vi "Module (Top Level).vi"(8 "error in":errorcluster) -> (0 "error out":errorcluster)   [LabVIEW 2017, in "Logger.lvlib"]
uses:
  Logger.lvlib
  User Events/TypeDefs/Shutdown UE FGV Command.ctl
  Global TypeDefs/Registered Modules.ctl
  Private TypeDefs/Messages.ctl
  Error Handler/Error Handler.lvlib
panel:
  out "Log (temporary)":string
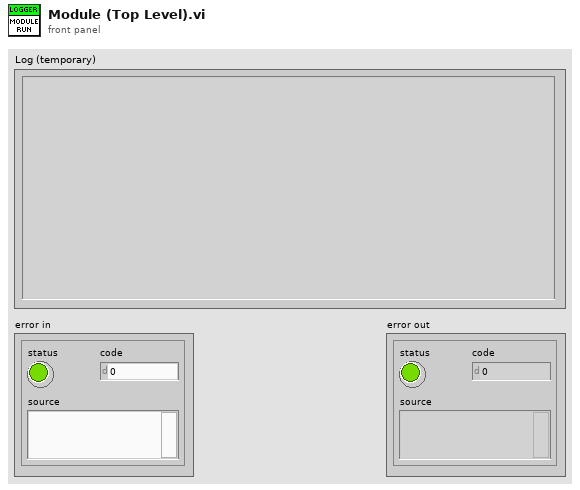
[diagram p1: front panel]
types:
  T1 = typedef "Registered Modules.ctl" = enum16{"Controller", "DAQ", "Error Handler", "Game", "myPAM", "WinHost", "Logger"}
  T2 = typedef "Shutdown UE FGV Command.ctl" = enum16{"create", "get", "destroy"}
  T3 = typedef "Logger.lvlib/Module Reference.ctl" = cluster{"calling module":T1, "module queues":T4, "module notifiers":T5}
  T4 = typedef "Logger.lvlib/Module Queues.ctl" = cluster{"message queue":refnum<queue>}
  T5 = typedef "Logger.lvlib/Module Notifiers.ctl" = cluster{"dummy notifier":refnum<notifier>}
  T6 = typedef "Error Handler.lvlib/Module Reference.ctl" = cluster{"calling module":T1, "module queues":T7, "module notifiers":T8}
  T7 = typedef "Error Handler.lvlib/Module Queues.ctl" = cluster{"message queue":refnum<queue>}
  T8 = typedef "Error Handler.lvlib/Module Notifiers.ctl" = cluster{"dummy notifier":refnum<notifier>}
  T9 = enum16{"open", "replace", "create", "open or create", "replace or create", "replace or create with confirmation"}
  T10 = typedef "Logger.lvlib/Messages.ctl" = enum16{"log event", "shutdown"}
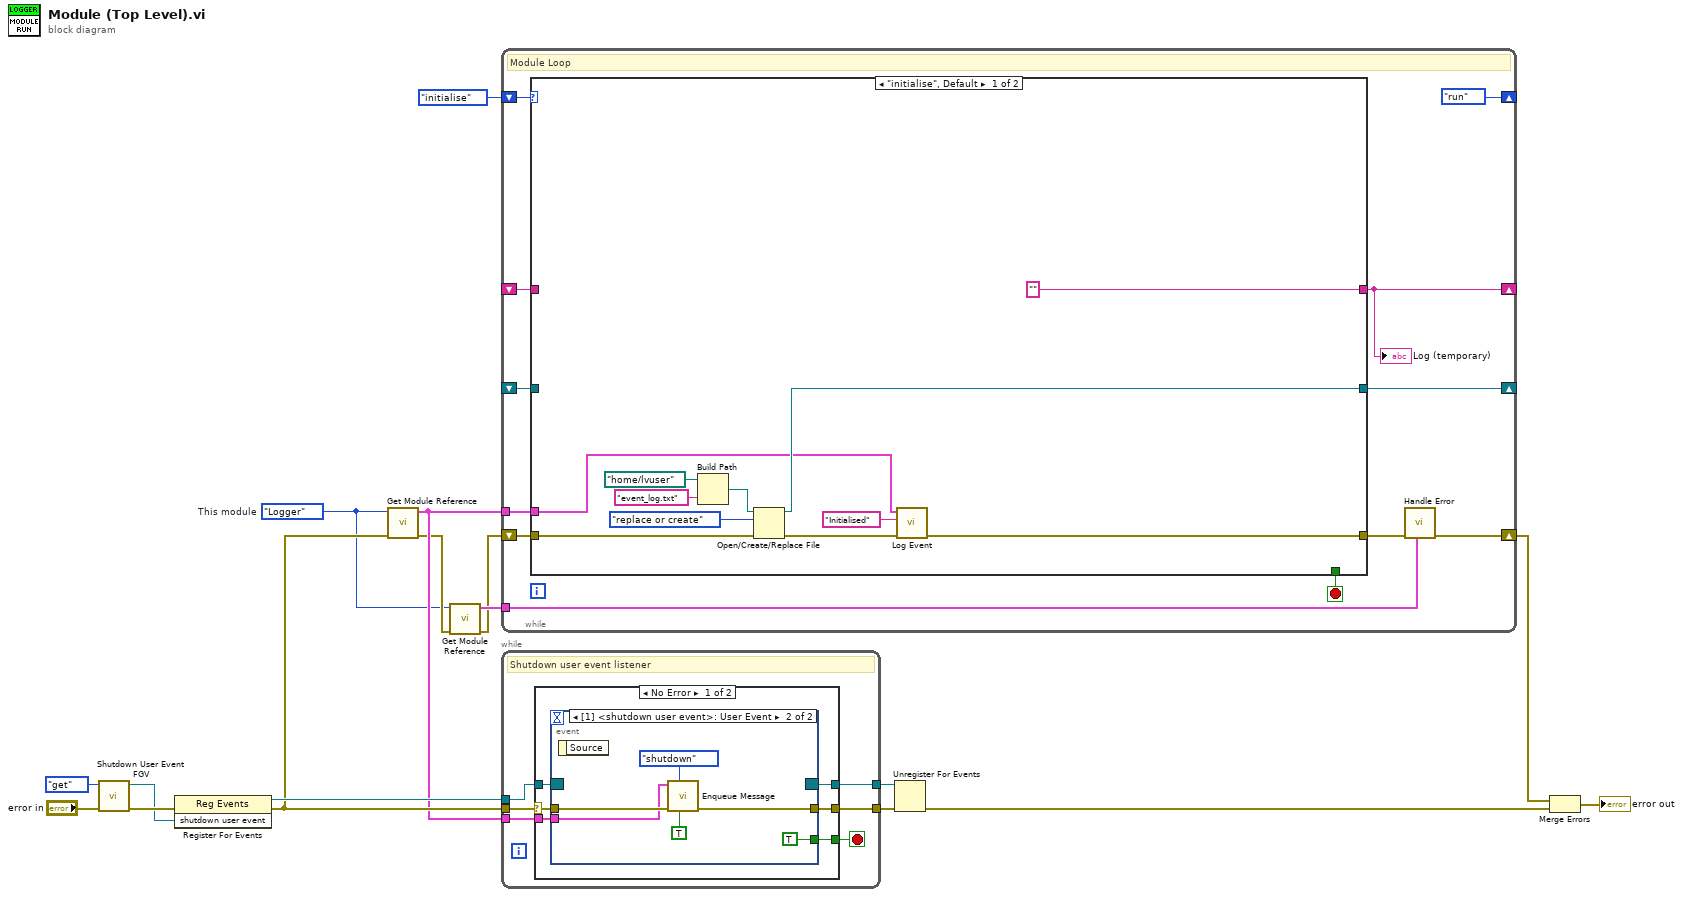
[diagram p0: block diagram]
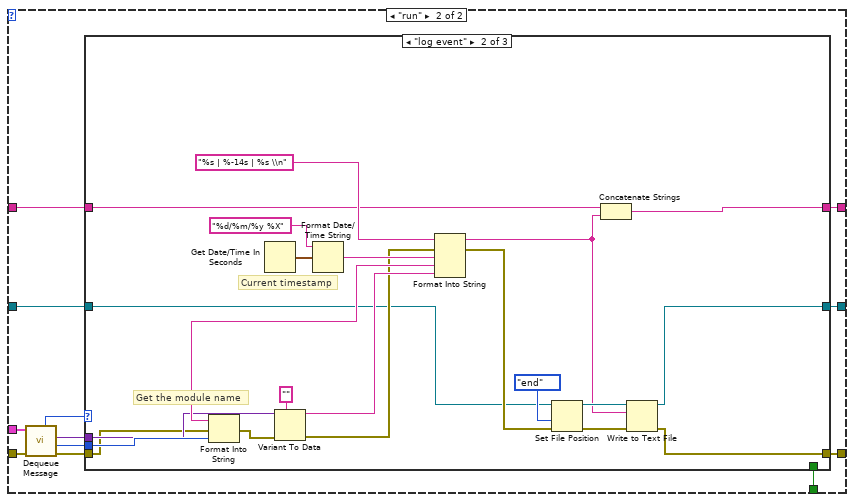
[diagram p2: hidden frame]
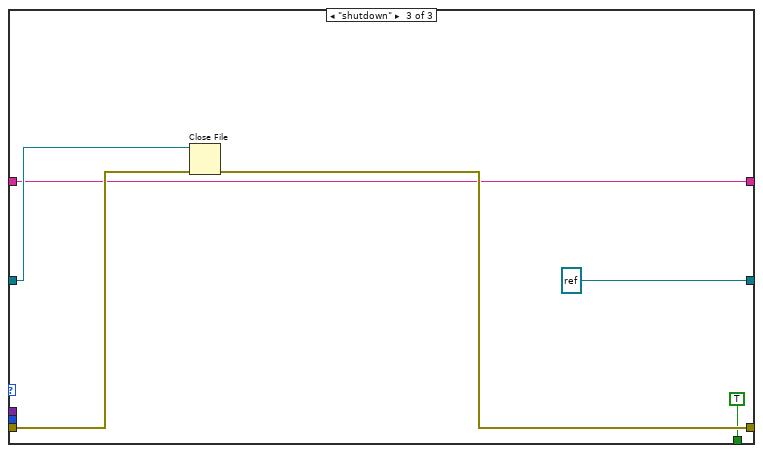
[diagram p4: hidden frame]
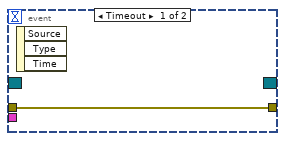
[diagram p5: hidden frame]
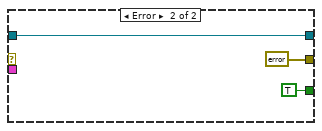
[diagram p6: hidden frame]
diagram:
  w3 = Registered_Modules."Logger"  # This module
  n1 = call "Shutdown User Event FGV.vi"("error in"="error in", "command"=Shutdown_UE_FGV_Command."get" ("Command")) -> ("error out"=w12:errorcluster, "shutdown user event"=w11:refnum<user-event>)  [unwired: 8 in]
  n2 = register-events(error in=w12, w11) -> (reference out=w16:refnum<event-registration>, error out=w7:errorcluster)  [unwired: 1 in]
  n3 = call "Get Module Reference.vi"("error in"=w7, "calling module"=w3) -> ("error out"=w4:errorcluster, "module reference"=w6:T3)  [unwired: 8 in]
  n4 = call "Get Module Reference.vi"("error in"=w4, "calling module"=w3) -> ("error out"=w1:errorcluster, "module reference"=w2:T6)  [unwired: 8 in]
  n5 = while {
    shift-right: [w20] -> w14
    shift-left: w1 -> [w22]
    tunnel: w6 -> [w29]
    shift-right: [w28] -> _
    shift-left: _ -> [w18]
    shift-right: [w24] -> _
    shift-left: _ -> [w27]
    shift-right: [enum16{"initialise", "run"}."run"] -> _
    shift-left: enum16{"initialise", "run"}."initialise" -> [w26]
    tunnel: w2 -> [w19]
    stop <- w23 stop-if-true
    # "Module Loop"
    n6 = case shown="\"initialise\", Default" w26 {
      tunnel: [w33 w52] -> w21
      tunnel: w29 -> [w32 w51]
      tunnel: [w34 w46] -> w28
      tunnel: w18 -> [_ w45]
      tunnel: ["" w43] -> w24
      tunnel: w27 -> [_ w44]
      tunnel: [_ w42] -> w23
      tunnel: w22 -> [w35 w41]
      frame "initialise", Default {
        n7 = Build Path(base path=path "/home/lvuser", name or relative path="event_log.txt") -> (appended path=w38:path)
        n8 = Open/Create/Replace File(file path (use dialog)=w38, error in=w35, operation (0:open)=T9."replace or create") -> (refnum out=w34:refnum<file>, error out=w37:errorcluster)  [unwired: 3 in, 1 out]
        n9 = call "Log Event.vi"("error in"=w37, "event"="Initialised", "module reference in"=w32) -> ("error out"=w33:errorcluster)  [unwired: 7 in, 1 out]
      }
      frame "run" {
        n10 = call "Dequeue Message.vi"("error in"=w41, "module reference in"=w51) -> ("error out"=w49:errorcluster, "source"=w47:T1, "data"=w48:variant, "message"=w50:T10)  [unwired: 5 in, 1 out]
        n11 = case shown="\"log event\"" w50 {
          tunnel: [w55 w57 w80] -> w52
          tunnel: w49 -> [w55 w61 w83]
          tunnel: w48 -> [_ w62 _]
          tunnel: w47 -> [_ w63 _]
          tunnel: [w54 w56 refnum<file> refnum ("refnum out")] -> w46
          tunnel: w45 -> [w54 w58 w82]
          tunnel: [w53 w60 w79] -> w43
          tunnel: w44 -> [w53 w59 w79]
          tunnel: [_ _ TRUE] -> w42
          frame Default {
          }
          frame "log event" {
            # "Get the module name"
            # "Current timestamp"
            n12 = Format Into String(error in=w61, w63) -> (resulting string=w69:string, error out=w71:errorcluster)  [unwired: 2 in]
            n13 = Get Date/Time In Seconds() -> (seconds since 1Jan1904=w76:timestamp)
            n14 = Variant To Data(error in=w71, type="", Variant=w62) -> (data=w68:string, error out=w67:errorcluster)
            n15 = Format Date/Time String(time format string (%c)="%d/%m/%y %X", seconds (now)=w76) -> (date/time string=w70:string)  [unwired: 1 in]
            n16 = Format Into String(format string="%s | %-14s | %s \\n", error in=w67, w70, w69, w68) -> (resulting string=w64:string, error out=w66:errorcluster)  [unwired: 1 in]
            n17 = Set File Position(refnum=w58, from (0:start)=enum16{"start", "end", "current"}."end", error in=w66) -> (refnum out=w72:refnum<file>, error out=w74:errorcluster)  [unwired: 1 in]
            n18 = Concatenate Strings(w59, w64) -> (w60:string)
            n19 = Write to Text File(file (use dialog)=w72, text=w64, error in=w74) -> (refnum out=w56:refnum<file>, error out=w57:errorcluster)  [unwired: 1 in, 1 out]
          }
          frame "shutdown" {
            n20 = Close File(refnum=w82, error in=w83) -> (error out=w80:errorcluster)  [unwired: 1 out]
          }
        }
      }
    }
    "Log (temporary)" <- w24
    n21 = call "Handle Error.vi"("module reference in"=w19, "error in"=w21) -> ("error out"=w20:errorcluster)  [unwired: 9 in]
  }
  n22 = while {
    tunnel: w16 -> [w89]
    tunnel: [w88] -> w15
    tunnel: w7 -> [w86]
    tunnel: [w85] -> w9
    tunnel: w6 -> [w84]
    stop <- w87 stop-if-true
    # "Shutdown user event listener"
    n23 = case shown="No Error" w86 {
      selector: w86 -> [w92 _]
      tunnel: w89 -> [w95 w104]
      tunnel: [w94 w104] -> w88
      tunnel: [w93 TRUE] -> w87
      tunnel: [w91 errorcluster {"status"=FALSE, "code"=0, "source"=""} ("error out")] -> w85
      tunnel: w84 -> [w90 _]
      frame No Error {
        n24 = event shown="[1] <shutdown user event>: User Event" {
          selector: w95 -> [_ _]
          dyn-events: [_ _] -> w94
          timeout: _ -> [_ _]
          tunnel: w92 -> [w96 w100]
          tunnel: [w96 w99] -> w91
          tunnel: [_ TRUE] -> w93
          tunnel: w90 -> [_ w98]
          event Timeout {
            n25 = event-data() -> ()  [unwired: 1 in, 3 out]
          }
          event User Event {
            n26 = event-data() -> ()  [unwired: 1 in, 1 out]
            n27 = call "Enqueue Message.vi"("high priority"=TRUE, "message"=Messages."shutdown", "error in"=w100, "module reference in"=w98) -> ("error out"=w99:errorcluster)  [unwired: 6 in, 1 out]
          }
        }
      }
      frame Error {
      }
    }
  }
  n28 = Unregister For Events(event registration refnum=w15, error in=w9) -> (error out=w10:errorcluster)
  n29 = Merge Errors(w14, w10) -> (→"error out":errorcluster)
